vi "Swerve Drive.vi"(0 "X":dbl(slide) scale=-1.0..1.0, 1 "Rot. Point X":dbl, 2 "Rot. Point Y":dbl, 7 "Y":dbl(slide)=-0.007874015748031496 scale=1.0..-1.0, 11 "Z":dbl(knob) scale=1.0..-1.0, 12 "Auto Controls":bool, 13 "Robot-Centric":bool=TRUE, 14 "Reset Gyro":bool) -> ()   [LabVIEW 2016]
uses:
  <vilib>/Rock Robotics/WPI/ThirdParty/CanMotor/TalonSRX/WPI_CANTalonSRX_APIControlMode.ctl
  <vilib>/Rock Robotics/WPI/ThirdParty/CanMotor/TalonSRX/WPI_CANTalonSRX_APIFeedbackSelect.ctl
  Apple Gyro/Apple Pi Gyro Library.lvlib
panel:
  in  "BR":bool
  in  "BL":bool
  in  "FR":bool
  in  "FL":bool
  in  "Debug?":bool
  in  "Reverse Output":bool
  in  "Reverse Sensor":bool=TRUE
  in  "PIDF":cluster{"P":dbl, "I":dbl, "D":dbl, "F":dbl}={"P"=0.8, "I"=0.0, "D"=0.0, "F"=0.0}
  in  "Gyro Select (Overide)":enum16{"IMU", "SPI", "Analog", "Navx"}(ring)=enum."Navx"
  in  "Override NT?":bool=TRUE
  in  "Robot Width":dbl=21.5
  in  "Deadband":dbl=0.04 format="%#_13g"
  in  "Robot Length":dbl=21.5
  # "Gyro"
  # "All Units in Inches"
  # "Use the Debug Function to turn off \nmodules individually. Only Active \nmodules will work in Debug Mode."
  # "SWERVE DRIVE\nVersion 4.0\n \nCory Lynch\nChris Garuti\nGavin Popkin\nApple Pi Robotics\nTeam 2067"
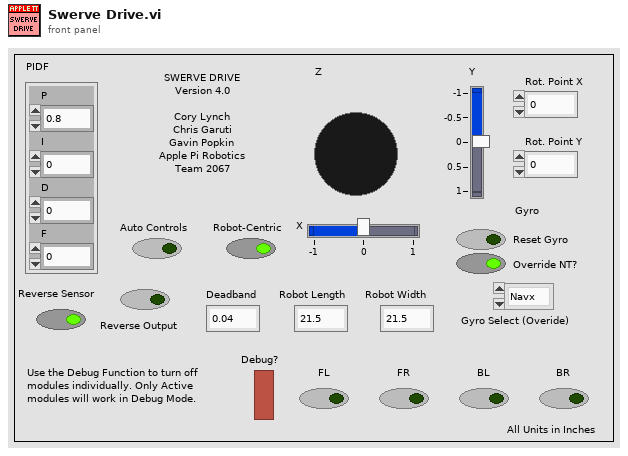
[diagram p1: front panel]
types:
  T1 = typedef "WPI_CANTalonSRX_APIFeedbackSelect.ctl" = enum16{"Digital Quadrature Encoder", "Analog Potentiometer", "Analog Encoder", "Count on Quad-A (Rising-Edge)", "Count on Quad-A (Falling-Edge)", "CTR Magnetic Enc (Absolute)", "CTR Magnetic Enc (Relative)", "Pulse Width"}
  T2 = typedef "WPI_MotorControlDeviceRef.ctl" = cluster{"DeviceStatus":errorcluster, "Type":T3, "PWM":cluster{"PWM Channel":T4, "DeadBand":T5}, "CAN":cluster{"Device Number":u8, "SetOutput VI Ref":variant, "GetOutput VI Ref":variant, "Enable VI Ref":variant, "Disable VI Ref":variant, "Data":variant}, "Invert":bool}
  T3 = typedef "WPI_MotorControlType.ctl" = enum16{"PWM", "CAN"}
  T4 = typedef "FPGA_DIOPWMChannel.ctl" = enum8{"PWM 0", "PWM 1", "PWM 2", "PWM 3", "PWM 4", "PWM 5", "PWM 6", "PWM 7", "PWM 8", "PWM 9", "PWM MXP 0", "PWM MXP 1", "PWM MXP 2", "PWM MXP 3", "PWM MXP 4", "PWM MXP 5", "PWM MXP 6", "PWM MXP 7", "PWM MXP 8", "PWM MXP 9", "Invalid"}
  T5 = typedef "WPI_PWMDeadband.ctl" = cluster{"Name":string, "maxPositivePwm":i32, "minPositivePwm":i32, "centerPwm":i32, "maxNegativePwm":i32, "minNegativePwm":i32, "angularRange":u16}
  T6 = typedef "WPI_CANTalonSRX_GlobalStatus.ctl" = cluster{"Applied Throttle":dbl, "Module Enabled":bool, "CAN Error":errorcluster, "Closed Loop Error":dbl, "Forward Limit Switch Closed":bool, "Reverse Limit Switch Closed":bool, "Sensor Position":dbl, "Sensor Velocity":dbl, "Current":dbl, "Sticky Fault - Over Temp":bool, "Sticky Fault - Under Voltage":bool, "Sticky Fault - Forward Limit":bool, "Sticky Fault - Reverse Limit":bool, "Sticky Fault - Forward Soft Limit":bool, "Sticky Fault - Reverse Soft Limit":bool, "Brake is Enabled":bool, "Encoder Position":dbl, "Encoder Velocity":dbl, "Encoder Index Count":dbl, "Encoder A Pin State":bool, "Encoder B Pin State":bool, "Encoder Index Pin State":bool, "Analog In":dbl, "Analog In Velocity":dbl, "Temperature (C)":dbl, "Battery Voltage":dbl, "Control 5 Is Supported":bool, "Current Profile Slot Select":dbl, "Pos Div 8":bool, "Vel Div 4":bool, "Pulse Width Position":i32, "Pulse Width Velocity":i32, "Pulse Width Rise To Rise (us)":i32, "Pulse Width Rise To Fall (us)":i32, "Mot Prof Active Is Under Run":bool, "Mot Prof Active Has Under Run":bool, "Mot Prof Active Is Last":bool, "Mot Prof Active Velocity Only":bool, "Mot Prof Active Is Valid":bool, "Mot Prof Buffer Is Full":bool, "Mot Prof Active Profile Slot Select":i32, "Mot Prof NextID":i32, "Mot Prof Count":i32, "Mot Prof Active Velocity":dbl, "Mot Prof Active Position":dbl, "Mot Prof Output Enable":i32}
  T7 = typedef "WPI_CANTalonSRX_APIControlMode.ctl" = enum8{"Percent VBus", "Speed", "Position", "Slave", "Unchanged / Invalid", "Voltage Compensation", "Current", "Motion Profile", "Motion Magic"}
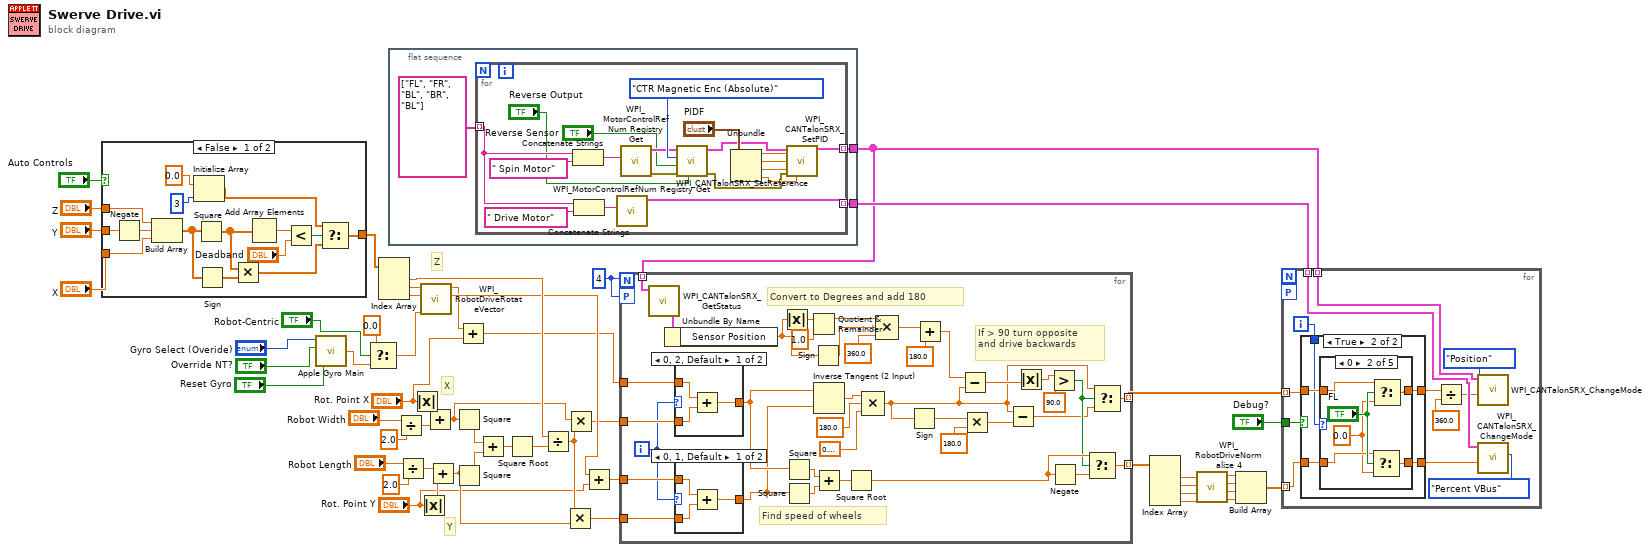
[diagram p0: block diagram]
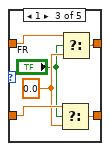
[diagram p4: hidden frame]
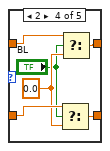
[diagram p5: hidden frame]
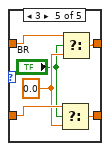
[diagram p6: hidden frame]
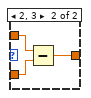
[diagram p7: hidden frame]
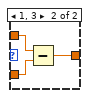
[diagram p8: hidden frame]
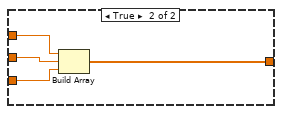
[diagram p9: hidden frame]
diagram:
  w18 = 4
  # "Z"
  # "X"
  # "Y"
  n1 = case shown="False" "Auto Controls" {
    tunnel: "Y" -> [w65 w71]
    tunnel: "X" -> [w59 w72]
    tunnel: "Z" -> [w55 w69]
    tunnel: [w56 w70] -> w47
    frame False {
      n2 = Negate(x=w65) -> (-x=w58:dbl)
      n3 = Build Array(w55, w58, w59) -> (w62:dbl[])
      n4 = Initialize Array(0.0 ("element"), 3 ("dimension size")) -> (w64:dbl[])
      n5 = Square(x=w62) -> (x^2=w60:dbl[])
      n6 = Sign(1:w62) -> (0:w61:dbl[])
      n7 = Multiply(x=w60, y=w61) -> (x*y=w57:dbl[])
      n8 = Add Array Elements(numeric array=w60) -> (sum=w68:dbl)
      n9 = Less?(x=w68, y="Deadband") -> (x < y?=w66:bool)
      n10 = Select(t=w64, s=w66, f=w57) -> (s? t:f=w56:dbl[])
    }
    frame True {
      n11 = Build Array(w69, w71, w72) -> (w70:dbl[])
    }
  }
  n12 = call "Apple Gyro Main.vi"("Reset Current"="Reset Gyro", "Override NT?"="Override NT?", "Gyro Select (Overide)"="Gyro Select (Overide)") -> ("Gyro Yaw Out"=w27:dbl)  [unwired: 1 in]
  n13 = Select(t=0.0, s="Robot-Centric", f=w27) -> (s? t:f=w46:dbl)
  n14 = Index Array(array=w47) -> (element #1=w44:dbl, element #2=w48:dbl, element #3=w51:dbl)  [unwired: 3 in]
  n15 = flat-sequence {
    tunnel: [w74] -> w17
    tunnel: [w73] -> w53
    frame #0 {
      n16 = for {
        tunnel: string[] ["FL", "FR", "BL", "BR", "BL"] -> [w85] mode=indexing
        tunnel: [w82] -> w74 mode=indexing
        tunnel: [w76] -> w73 mode=indexing
        n17 = Concatenate Strings(w85, " Spin Motor" ("refnum name")) -> (w84:string)
        n18 = Concatenate Strings(w85, " Drive Motor") -> (w83:string)
        n19 = call <vilib>:"WPI_MotorControlRefNum Registry Get.vi"("refnum name"=w83) -> ("MotorControlDevRef"=w76:T2)  [unwired: 9 in, 1 out]
        n20 = call <vilib>:"WPI_MotorControlRefNum Registry Get.vi"("refnum name"=w84) -> ("error out"=w80:errorcluster, "MotorControlDevRef"=w88:T2)  [unwired: 9 in]
        n21 = call <vilib>:"WPI_CANTalonSRX_SetReference.vi"("Reverse Closed-Loop Output"="Reverse Output", "error in (no error)"=w80, "Reverse Feedback Sensor"="Reverse Sensor", "Feedback Reference"=WPI_CANTalonSRX_APIFeedbackSelect."CTR Magnetic Enc (Absolute)", "CAN Talon SRX Ref"=w88) -> ("error out"=w79:errorcluster, "CAN Talon SRX Ref"=w89:T2)  [unwired: 5 in]
        n22 = Unbundle("PIDF") -> ("P"=w90:dbl, "I"=w92:dbl, "D"=w91:dbl, "F"=w81:dbl)
        n23 = call <vilib>:"WPI_CANTalonSRX_SetPID.vi"("CAN Talon SRX Ref"=w89, "P"=w90, "I"=w92, "D"=w91, "error in (no error)"=w79, "F"=w81) -> ("CAN Talon SRX Ref"=w82:T2)  [unwired: 8 in, 1 out]
      }
    }
  }
  n24 = Divide(x="Robot Width", y=2.0) -> (x/y=w13:dbl)
  n25 = Divide(x="Robot Length", y=2.0) -> (x/y=w12:dbl)
  n26 = Absolute Value(x="Rot. Point X") -> (abs(x)=w14:dbl)
  n27 = Absolute Value(x="Rot. Point Y") -> (abs(x)=w11:dbl)
  n28 = call <vilib>:"WPI_RobotDriveRotateVector.vi"("Angle"=w46, "X"=w51, "Y"=w48) -> ("X'"=w42:dbl, "Y'"=w41:dbl)  [unwired: 7 out]
  n29 = Add(x=w14, y=w13) -> (x+y=w16:dbl)
  n30 = Add(x=w12, y=w11) -> (x+y=w15:dbl)
  n31 = Square(x=w16) -> (x^2=w24:dbl)
  n32 = Square(x=w15) -> (x^2=w21:dbl)
  n33 = Add(x=w41, y="Rot. Point X") -> (x+y=w5:dbl)
  n34 = Add(x=w24, y=w21) -> (x+y=w25:dbl)
  n35 = Square Root(x=w25) -> (sqrt(x)=w19:dbl)
  n36 = Divide(x=w44, y=w19) -> (x/y=w43:dbl)
  n37 = Multiply(x=w43, y=w15) -> (x*y=w39:dbl)
  n38 = Multiply(x=w16, y=w43) -> (x*y=w40:dbl)
  n39 = Add(x=w42, y="Rot. Point Y") -> (x+y=w3:dbl)
  n40 = for {
    N: w18 -> [_]
    tunnel: w5 -> [w131]
    tunnel: w40 -> [w130]
    tunnel: w3 -> [w129]
    tunnel: w39 -> [w128]
    tunnel: [w95] -> w6 mode=indexing
    tunnel: [w96] -> w7 mode=indexing
    tunnel: w17 -> [w120] mode=indexing
    workers-P: w18 -> [_]
    i -> [w99]
    # "Find speed of wheels"
    # "If > 90 turn opposite \nand drive backwards"
    # "Convert to Degrees and add 180"
    n41 = call <vilib>:"WPI_CANTalonSRX_GetStatus.vi"("CAN Talon SRX Ref"=w120) -> ("Talon SRX Status"=w119:T6)  [unwired: 8 in, 2 out]
    n42 = Unbundle By Name(w119) -> ("Sensor Position"=w116:dbl)
    n43 = case shown="0, 2, Default" w99 {
      tunnel: w131 -> [w140 w143]
      tunnel: w130 -> [w139 w142]
      tunnel: [w138 w141] -> w98
      frame 0, 2, Default {
        n44 = Add(x=w140, y=w139) -> (x+y=w138:dbl)
      }
      frame 1, 3 {
        n45 = Subtract(x=w143, y=w142) -> (x-y=w141:dbl)
      }
    }
    n46 = case shown="0, 1, Default" w99 {
      tunnel: w129 -> [w134 w137]
      tunnel: w128 -> [w133 w136]
      tunnel: [w132 w135] -> w97
      frame 0, 1, Default {
        n47 = Add(x=w134, y=w133) -> (x+y=w132:dbl)
      }
      frame 2, 3 {
        n48 = Subtract(x=w137, y=w136) -> (x-y=w135:dbl)
      }
    }
    n49 = Absolute Value(x=w116) -> (abs(x)=w117:dbl)
    n50 = Square(x=w98) -> (x^2=w125:dbl)
    n51 = Square(x=w97) -> (x^2=w126:dbl)
    n52 = Quotient & Remainder(x=w117, y=1.0) -> (x-y*floor(x/y)=w113:dbl)  [unwired: 1 out]
    n53 = Sign(1:w116) -> (0:w111:dbl)
    n54 = Inverse Tangent (2 Input)(1:w97, 2:w98) -> (0:w127:dbl)
    n55 = Add(x=w125, y=w126) -> (x+y=w124:dbl)
    n56 = Square Root(x=w124) -> (sqrt(x)=w121:dbl)
    n57 = Compound Arithmetic op=MULTIPLY(w127, 180.0, 0.3183098861837907) -> (w103:dbl)
    n58 = Compound Arithmetic op=MULTIPLY(w113, w111, 360.0 ("y")) -> (w115:dbl)
    n59 = Sign(1:w103) -> (0:w106:dbl)
    n60 = Add(x=w115, y=180.0) -> (x+y=w110:dbl)
    n61 = Subtract(x=w110, y=w103) -> (x-y=w105:dbl)
    n62 = Multiply(x=w106, y=180.0) -> (x*y=w107:dbl)
    n63 = Subtract(x=w103, y=w107) -> (x-y=w104:dbl)
    n64 = Absolute Value(x=w105) -> (abs(x)=w101:dbl)
    n65 = Greater?(x=w101, y=90.0 ("lower limit")) -> (0:w114:bool)
    n66 = Negate(x=w121) -> (-x=w123:dbl)
    n67 = Select(t=w121, s=w114, f=w123) -> (s? t:f=w95:dbl)
    n68 = Select(t=w103, s=w114, f=w104) -> (s? t:f=w96:dbl)
  }
  n69 = Index Array(array=w6) -> (element #1=w38:dbl, element #2=w37:dbl, element #3=w36:dbl, element #4=w35:dbl)  [unwired: 4 in]
  n70 = call <vilib>:"WPI_RobotDriveNormalize 4.vi"("D"=w35, "C"=w36, "B"=w37, "A"=w38) -> ("D'"=w31:dbl, "C'"=w32:dbl, "B'"=w33:dbl, "A'"=w34:dbl)
  n71 = Build Array(w34, w33, w32, w31) -> (w30:dbl[])
  n72 = for {
    tunnel: w7 -> [w148] mode=indexing
    tunnel: w17 -> [w154] mode=indexing
    tunnel: w53 -> [w152] mode=indexing
    tunnel: w30 -> [w149] mode=indexing
    workers-P: _ -> [_]
    tunnel: "Debug?" -> [w144]
    i -> [w145]
    n73 = case shown="True" w144 {
      tunnel: [w157 w162] -> w147
      tunnel: w148 -> [w157 w160]
      tunnel: w149 -> [w156 w159]
      tunnel: [w156 w161] -> w146
      tunnel: w145 -> [_ w158]
      frame False {
      }
      frame True {
        n74 = case shown="0" w158 {
          tunnel: [w164 w170 w176 w182 w188] -> w162
          tunnel: [w163 w169 w175 w181 w187] -> w161
          tunnel: w160 -> [w164 w167 w174 w180 w186]
          tunnel: w159 -> [w163 w166 w173 w179 w185]
          frame -1, Default {
            # "It forced me to make a default case that will never happen"
          }
          frame 0 {
            w165 = 0.0 ("t")
            n75 = Select(t=w166, s="FL", f=w165) -> (s? t:f=w169:dbl)
            n76 = Select(t=w167, s="FL", f=w165) -> (s? t:f=w170:dbl)
          }
          frame 1 {
            w172 = 0.0 ("t")
            n77 = Select(t=w173, s="FR", f=w172) -> (s? t:f=w175:dbl)
            n78 = Select(t=w174, s="FR", f=w172) -> (s? t:f=w176:dbl)
          }
          frame 2 {
            w178 = 0.0 ("t")
            n79 = Select(t=w179, s="BL", f=w178) -> (s? t:f=w181:dbl)
            n80 = Select(t=w180, s="BL", f=w178) -> (s? t:f=w182:dbl)
          }
          frame 3 {
            w184 = 0.0 ("t")
            n81 = Select(t=w185, s="BR", f=w184) -> (s? t:f=w187:dbl)
            n82 = Select(t=w186, s="BR", f=w184) -> (s? t:f=w188:dbl)
          }
        }
      }
    }
    n83 = Divide(x=w147, y=360.0) -> (x/y=w151:dbl)
    n84 = call <vilib>:"WPI_CANTalonSRX_ChangeMode.vi"("Output"=w151, "Control Mode"=WPI_CANTalonSRX_APIControlMode."Position", "CAN Talon SRX Ref"=w154) -> ()  [unwired: 7 in, 2 out]
    n85 = call <vilib>:"WPI_CANTalonSRX_ChangeMode.vi"("Output"=w146, "Control Mode"=WPI_CANTalonSRX_APIControlMode."Percent VBus", "CAN Talon SRX Ref"=w152) -> ()  [unwired: 7 in, 2 out]
  }
